vi "Generate Test Event.vi"(8 "error in (no error)":errorcluster, 11 "Timing Engine Tester in":refnum<class "Timing Engine Tester.lvclass">) -> (0 "error out":errorcluster, 3 "Timing Engine Tester out":refnum<class "Timing Engine Tester.lvclass">)   [LabVIEW 2016, in "Assert API Components.lvlib" / "Assert Display.lvlib" / "Timing Engine Tester.lvlib" / "Timing Engine Tester.lvclass"]
uses:
  Timing Engine Tester.lvclass
  Timing Engine Tester.lvclass/Timing Engine Tester.ctl
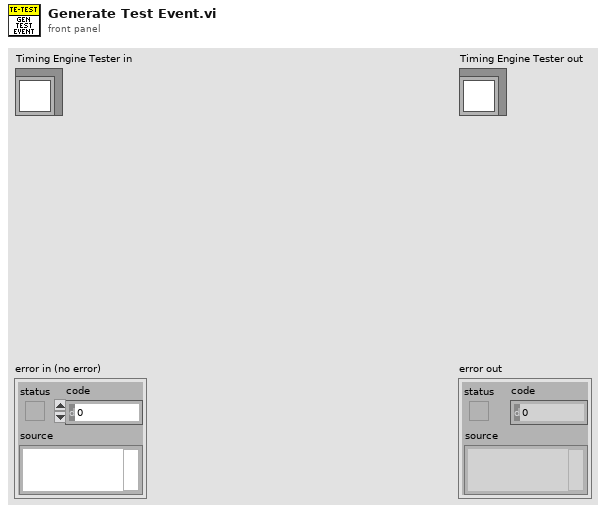
[diagram p1: front panel]
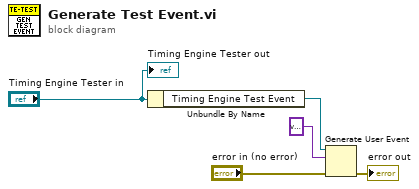
[diagram p0: block diagram]
diagram:
  n1 = Unbundle By Name("Timing Engine Tester in") -> ("Timing Engine Test Event"=w4:refnum<user-event>)
  n2 = Generate User Event(user event=w4, event data cluster=variant ("event data"), error in="error in (no error)") -> (error out=→"error out":errorcluster)  [unwired: 1 in, 1 out]
  "Timing Engine Tester out" <- "Timing Engine Tester in"
